vi "Cvt CellPos to Bounds.vi"(10 "CellPosition":T2, 11 "D_Datagrid in":refnum<class "D_Datagrid.lvclass">) -> (3 "Bounds":T1)   [LabVIEW 2018]
doc: "Converts a cell position (row/column) to pixel bounds."
uses:
  D_Datagrid.lvclass
  C:/Program Files (x86)/National Instruments/LabVIEW 2018/vi.lib/QSI/QControls/QControl Classes/Table/Table.lvclass
  C:/Program Files (x86)/National Instruments/LabVIEW 2018/vi.lib/QSI/QControls/QControl Classes/Control/Control.lvclass
  <vilib>/Utility/miscctls.llb/LVRowAndColumnTypeDef.ctl
  <vilib>/Utility/miscctls.llb/LVRectTypeDef.ctl
  <vilib>/Utility/miscctls.llb/LVPointTypeDef.ctl
  D_Datagrid.lvclass/D_Datagrid.ctl
  Read Top level parent.vi
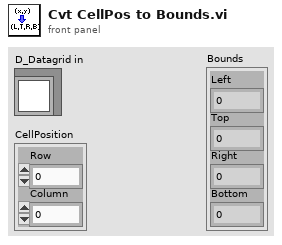
[diagram p1: front panel]
types:
  T1 = typedef "LVRectTypeDef.ctl" = cluster{"Left":i16, "Top":i16, "Right":i16, "Bottom":i16}
  T2 = typedef "LVRowAndColumnTypeDef.ctl" = cluster{"Row":i32, "Column":i32}
  T3 = typedef "LVPointTypeDef.ctl" = cluster{"Horizontal":i16, "Vertical":i16}
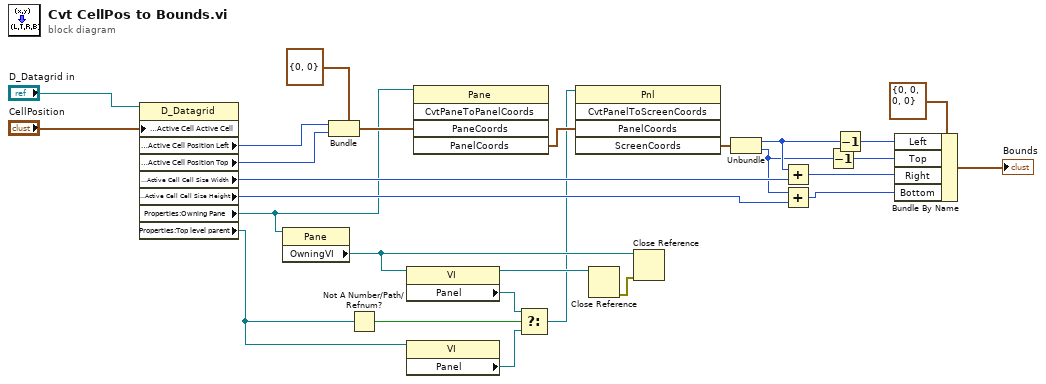
[diagram p0: block diagram]
diagram:
  n1 = property class="D_Datagrid"(reference="D_Datagrid in", "Properties:Active Cell Active Cell"="CellPosition") -> ("Properties:Active Cell Position Left"=w20:i32, "Properties:Active Cell Position Top"=w22:i32, "Properties:Active Cell Cell Size Width"=w25:u32, "Properties:Active Cell Cell Size Height"=w26:u32, "Properties:Owning Pane"=w19:refnum<vi>, "Properties:Top level parent"=w2:refnum<vi>)  [unwired: 1 in, 2 out]
  n2 = property class="Pane"(reference=w19) -> ("OwningVI"=w18:refnum<vi>)  [unwired: 1 in, 2 out]
  n3 = Bundle(cluster=T3 {"Horizontal"=0, "Vertical"=0} ("Pane Coordinates"), "Horizontal"=w20, "Vertical"=w22) -> (w21:T3)
  n4 = Not A Number/Path/Refnum?(number/path/refnum=w2) -> (NaN/Path/Refnum?=w5:bool)
  n5 = property class="VI"(reference=w18) -> (reference out=w24:refnum<vi>, "Panel"=w4:refnum<vi>)  [unwired: 1 in, 1 out]
  n6 = property class="VI"(reference=w2) -> ("Panel"=w1:refnum<vi>)  [unwired: 1 in, 2 out]
  n7 = invoke class="Pane" method="CvtPaneToPanelCoords"(reference=w19, "PaneCoords"=w21) -> ("PanelCoords"=w14:T3)  [unwired: 3 in, 4 out]
  n8 = Select(t=w4, s=w5, f=w1) -> (s? t:f=w3:refnum<vi>)
  n9 = invoke class="Pnl" method="CvtPanelToScreenCoords"(reference=w3, "PanelCoords"=w14) -> ("ScreenCoords"=w13:T3)  [unwired: 3 in, 4 out]
  n10 = Close Reference(reference=w24) -> (error out=w15:errorcluster)  [unwired: 1 in]
  n11 = Close Reference(reference=w18, error in (no error)=w15) -> ()  [unwired: 1 out]
  n12 = Unbundle(w13) -> ("Horizontal"=w12:i16, "Vertical"=w11:i16)
  n13 = Add(x=w12, y=w25) -> (x+y=w17:u32)
  n14 = Add(x=w11, y=w26) -> (x+y=w16:u32)
  n15 = Decrement(x=w11) -> (x-1=w6:i16)
  n16 = Decrement(x=w12) -> (x-1=w7:i16)
  n17 = Bundle By Name(cluster=T1 {"Left"=0, "Top"=0, "Right"=0, "Bottom"=0} ("Bounds"), "Left"=w7, "Top"=w6, "Right"=w17, "Bottom"=w16) -> (→"Bounds":T1)
